vi "Add Parameter Channels with Definitions.vi"(6 "direction":T4, 8 "error in":errorcluster, 10 "parameters":T3(array[cluster]), 11 "message or subaddress":T1 format="%.0x") -> (0 "error out":errorcluster, 3 "message or subaddress out":T1 format="%.0x")   [LabVIEW 2020, in "AIM MIL-STD-1553 Scripting.lvlib"]
doc: "Sets the direction of the <b>message or subaddress</b>, and then adds a new channel to the <b>message or subaddress</b> section for each element in <b>parameters</b>."
uses:
  AIM MIL-STD-1553 Scripting.lvlib
  Shared/Direction.ctl
  <vilib>/NI VeriStand/Custom Device API/Custom Device Item Ref.ctl
  Shared/Parameter Definition.ctl
  <vilib>/NI VeriStand/Custom Device API/Custom Device Channel Type.ctl
  <vilib>/NI VeriStand/Custom Device API/Custom Device Channel.ctl
  <vilib>/NI VeriStand/Custom Device API/Custom Device API.lvlib
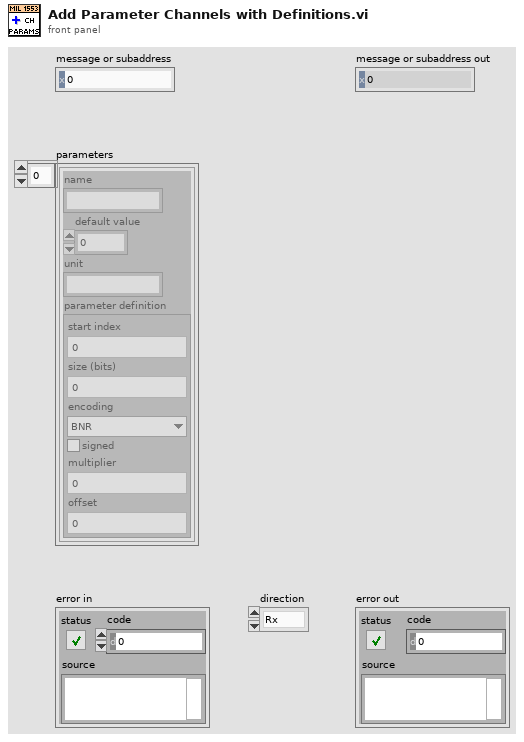
[diagram p1: front panel]
types:
  T1 = typedef "Custom Device API.lvlib/Custom Device Item Ref.ctl" = u64
  T2 = typedef "Parameter Definition.ctl" = cluster{"start index":i32, "size (bits)":i32, "encoding":enum16{"BNR", "BCD", "Discrete"}, "signed":bool, "multiplier":dbl, "offset":dbl}
  T3 = cluster{"name":string, "default value":dbl, "unit":string, "parameter definition":T2}[]
  T4 = typedef "Direction.ctl" = enum16{"Rx", "Tx"}
  T5 = typedef "Custom Device API.lvlib/Custom Device Channel Type.ctl" = enum16{"Input", "Output"}
  T6 = typedef "Custom Device API.lvlib/Custom Device Channel.ctl" = cluster{"Type":T5, "Units":string, "Default Value":dbl, "Faultable":bool, "Scalable":bool}
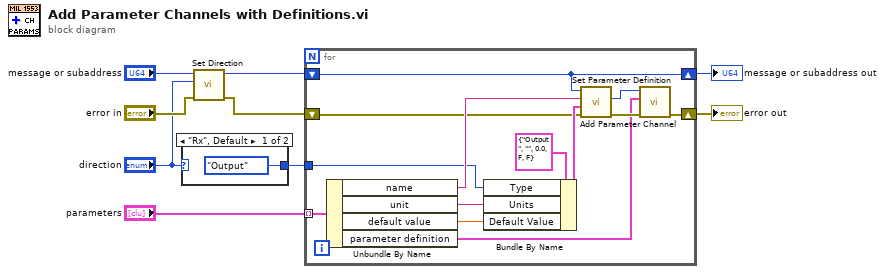
[diagram p0: block diagram]
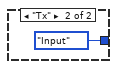
[diagram p2: hidden frame]
diagram:
  n1 = case shown="\"Rx\", Default" "direction" {
    tunnel: [Custom_Device_Channel_Type."Output" ("Type") Custom_Device_Channel_Type."Input" ("Type")] -> w6
    frame "Rx", Default {
    }
    frame "Tx" {
    }
  }
  n2 = call "Set Direction.vi"("error in"="error in", "direction"="direction", "message or subaddress"="message or subaddress") -> ("error out"=w2:errorcluster, "message or subaddress out"=w4:T1)  [unwired: 7 in]
  n3 = for {
    shift-right: [w16] -> w9
    shift-left: w4 -> [w16]
    tunnel: "parameters" -> [w24] mode=indexing
    shift-right: [w14] -> w8
    shift-left: w2 -> [w15]
    tunnel: w6 -> [w13]
    n4 = Unbundle By Name(w24) -> ("name"=w20:string, "unit"=w22:string, "default value"=w21:dbl, "parameter definition"=w17:T2)
    n5 = Bundle By Name(cluster=T6 {"Type"=enum."Output", "Units"="", "Default Value"=0.0, "Faultable"=FALSE, "Scalable"=FALSE} ("Channel"), "Type"=w13, "Units"=w22, "Default Value"=w21) -> (w19:T6)
    n6 = call "Add Parameter Channel.vi"("error in"=w15, "channel definition"=w19, "name"=w20, "section"=w16) -> ("error out"=w18:errorcluster, "channel"=w12:T1)  [unwired: 5 in, 1 out]
    n7 = call "Set Parameter Definition.vi"("error in"=w18, "parameter definition"=w17, "parameter"=w12) -> ("error out"=w14:errorcluster)  [unwired: 7 in, 1 out]
  }
  "message or subaddress out" <- w9
  "error out" <- w8
